vi "lab3.vi"() -> ()   [LabVIEW 2015]
uses:
  <vilib>/Analysis/polynomials.llb/Scalar Polynomial Evaluation (DBL).vi
  <vilib>/ptbypt/NI_PtbyPt.lvlib
  <vilib>/Analysis/NI_AALPro.lvlib
panel:
  out "Waveform Chart":dynamicdata(graph)
  in  "P(x)":dbl[](array[numeric])=[8.0, -2.0, 0.02] format="%#.10f"
  in  "stop":bool
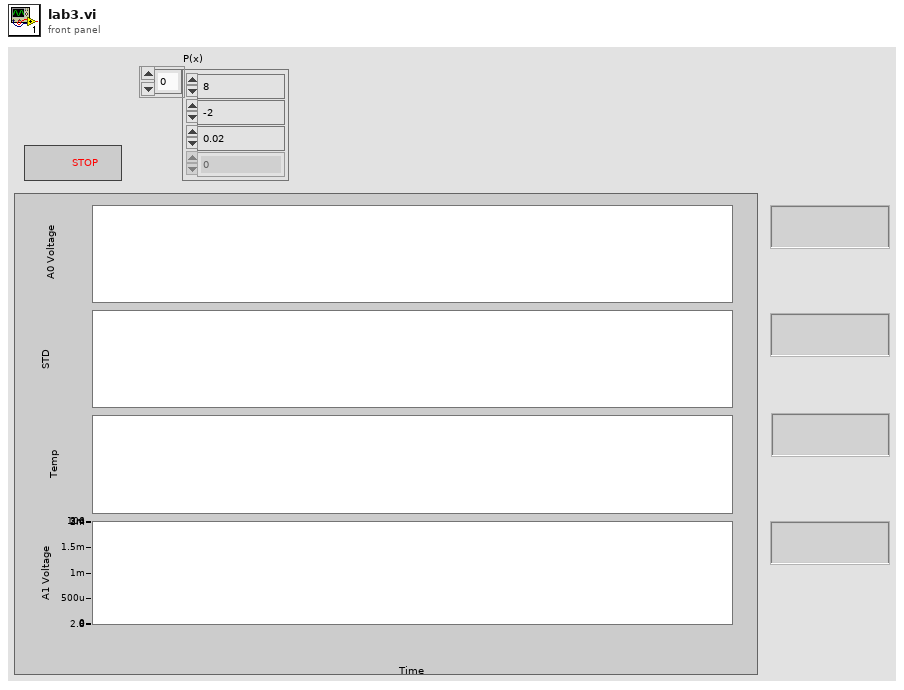
[diagram p1: front panel]
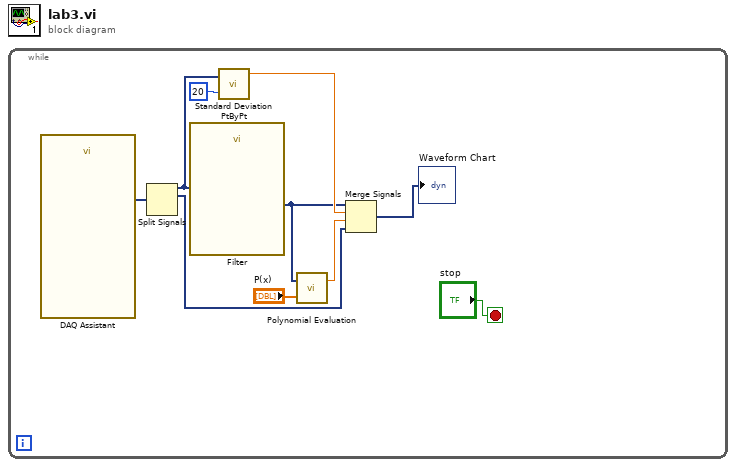
[diagram p0: block diagram]
diagram:
  n1 = while {
    stop <- "stop" stop-if-true
    n2 = call "DAQ Assistant"() -> ("data"=w6:dynamicdata)  [unwired: 17 in, 2 out]
    n3 = Split Signals(w6) -> (w4:dynamicdata, w2:dynamicdata)  [unwired: 4 in, 2 out]
    n4 = call "Filter"("Signal"=w4) -> ("Filtered Signal"=w3:dynamicdata)  [unwired: 9 in, 1 out]
    n5 = call <vilib>:"Standard Deviation PtByPt.vi"("x"=w4, "sample length"=20) -> ("standard deviation"=w10:dbl)  [unwired: 1 in, 2 out]
    n6 = call-poly <vilib>:"Polynomial Evaluation.vi"("P(x)"="P(x)", "a"=w3) -> ("P(a)"=w5:dbl)  [unwired: 1 out]
    n7 = Merge Signals(w3, w10, w5, w2) -> (→"Waveform Chart":dynamicdata)
  }
